vi "OffsetCalculatorCore.vi"(2 "VertOffsetFormula":string, 3 "HorzOffsetFormula":string, 4 "Distance":dbl[](array[numeric])) -> (0 "VertOffset":dbl[](array[numeric]), 1 "HorzOffset":dbl[](array[numeric]))   [LabVIEW 2012]
uses:
  <vilib>/gmath/NI_Gmath.lvlib
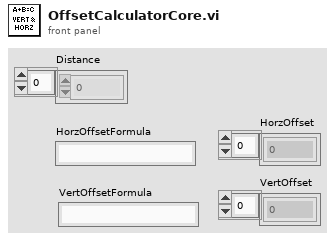
[diagram p1: front panel]
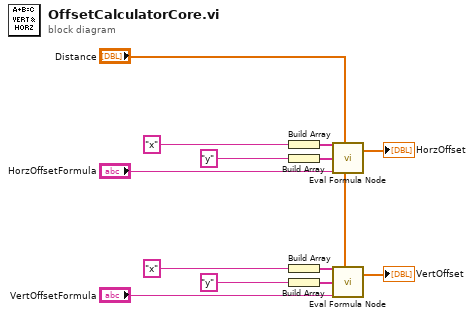
[diagram p0: block diagram]
diagram:
  n1 = Build Array("x") -> (w9:string[])
  n2 = Build Array("y") -> (w8:string[])
  n3 = Build Array("x") -> (w3:string[])
  n4 = Build Array("y") -> (w2:string[])
  n5 = call <vilib>:"Eval Formula Node.vi"("Variables Input"=w9, "Input Values"="Distance", "Variables Output"=w8, "formula"="HorzOffsetFormula") -> ("Output Values"=→"HorzOffset":dbl[])  [unwired: 1 in, 1 out]
  n6 = call <vilib>:"Eval Formula Node.vi"("Variables Input"=w3, "Input Values"="Distance", "Variables Output"=w2, "formula"="VertOffsetFormula") -> ("Output Values"=→"VertOffset":dbl[])  [unwired: 1 in, 1 out]
